vi "Plugin ID to Tree Items.vi"(8 "error in (no error)":errorcluster, 9 "Plugin ID":string, 11 "Application Data in":T2) -> (0 "error out":errorcluster, 1 "Settings":T1, 2 "Item":T1, 3 "Application Data out":T2)   [LabVIEW 2017, in "DSF Configuration Utility.lvlib"]
uses:
  DSF Configuration Utility.lvlib
  Main VI/Application Data.ctl
  VeriStand/Data Sharing Custom Device/Source/DSF Core.lvlibp/Classes/Configuration/Configuration Session.lvclass
  Main VI/View Mode.ctl
  Tree Item.ctl
  Tree Item Type.ctl
  VeriStand/Data Sharing Custom Device/Source/DSF Core.lvlibp/Classes/Configuration/Read Settings.vi
  VeriStand/Data Sharing Custom Device/Source/DSF Core.lvlibp/Classes/Configuration/Read Plugin.vi
panel:
  # "App\nData"
  # "App\nData"
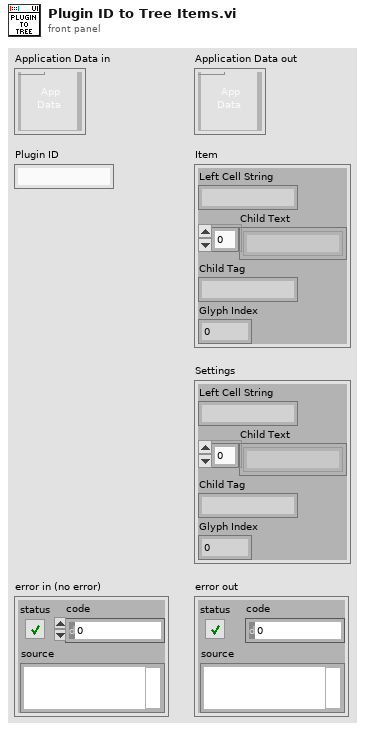
[diagram p1: front panel]
types:
  T1 = typedef "DSF Configuration Utility.lvlib/Tree Item.ctl" = cluster{"Left Cell String":string, "Child Text":string[], "Child Tag":string, "Glyph Index":i32}
  T2 = typedef "DSF Configuration Utility.lvlib/Application Data.ctl" = cluster{"Item Tree Control":refnum<vi>, "Value Tree Control":refnum<vi>, "DSF Refnum":refnum<class "Configuration Session.lvclass">, "Top-Level VI":refnum<vi>, "View State":T3, "menu reference":refnum<k9>}
  T3 = typedef "DSF Configuration Utility.lvlib/View Mode.ctl" = enum16{"Tree", "List"}
  T4 = typedef "DSF Configuration Utility.lvlib/Tree Item Type.ctl" = enum16{"Plugin", "Group", "Transfer", "Channel", "Setting"}
  T5 = typedef "DSF Core.lvlibp/DSF Plugin Info.ctl" = cluster{"components":string[], "timing":T6, "group ids":string[], "settings id":string, "threads":T7[]}
  T6 = typedef "DSF Core.lvlibp/DSF Timing Info.ctl" = cluster{"priority":u64, "decimation":u64, "offset":u64}
  T7 = typedef "DSF Core.lvlibp/DSF Engine Plugin Thread Configuration.ctl" = cluster{"buffer converter settings":T8, "transceiver settings":T8, "custom settings":T8, "processor":i32, "priority offset":i16}
  T8 = typedef "DSF Core.lvlibp/DSF Settings Info.ctl" = cluster{"key":string, "value":string}[]
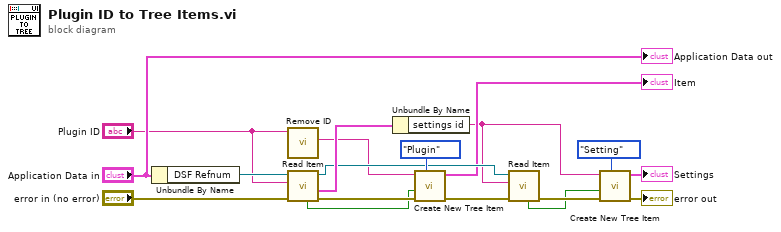
[diagram p0: block diagram]
diagram:
  n1 = Unbundle By Name("Application Data in") -> ("DSF Refnum"=w10:refnum<class "Configuration Session.lvclass">)
  n2 = call "Remove ID.vi"("id string"="Plugin ID") -> ("name"=w1:string)  [unwired: 8 in, 2 out]
  n3 = call-poly "Read Item.vi"("error in (no error)"="error in (no error)", "Plugin ID"="Plugin ID", "Configuration Session in"=w10) -> ("error out"=w13:errorcluster, "value"=w15:T5, "Configuration Session out"=w9:refnum<class "Configuration Session.lvclass">, "found?"=w4:bool)  [unwired: 5 in]
  n4 = Unbundle By Name(w15) -> ("settings id"=w3:string)
  n5 = call "Create New Tree Item.vi"("Item Type"=Tree_Item_Type."Plugin", "error in"=w13, "found?"=w4, "Left Cell String"=w1) -> ("error out"=w12:errorcluster, "Item"=→"Item":T1)  [unwired: 6 in]
  n6 = call-poly "Read Item.vi"("error in (no error)"=w12, "Settings ID"=w3, "Configuration Session in"=w9) -> ("error out"=w16:errorcluster, "found?"=w5:bool)  [unwired: 5 in, 2 out]
  n7 = call "Create New Tree Item.vi"("Item Type"=Tree_Item_Type."Setting", "error in"=w16, "found?"=w5, "Left Cell String"=w3) -> ("error out"=→"error out":errorcluster, "Item"=→"Settings":T1)  [unwired: 6 in]
  "Application Data out" <- "Application Data in"
